vi "Autoscale_Y.vi"   [LabVIEW 2012]
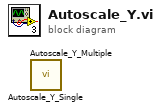
[diagram p0: block diagram]
diagram:
  n1 = call "Autoscale_Y_Single.vi"() -> ()  [unwired: 12 in]
  n2 = call "Autoscale_Y_Multiple.vi"() -> ()  [unwired: 12 in]
